vi "INIT.vi"(8 "error in (no error)":errorcluster, 11 "STREAK_camera in":refnum<class "STREAK_camera.lvclass">) -> (0 "error out":errorcluster, 3 "STREAK_camera out":refnum<class "STREAK_camera.lvclass">)   [LabVIEW 2019, in "STREAK_camera.lvclass"]
uses:
  STREAK_camera.lvclass
  Detector.lvclass
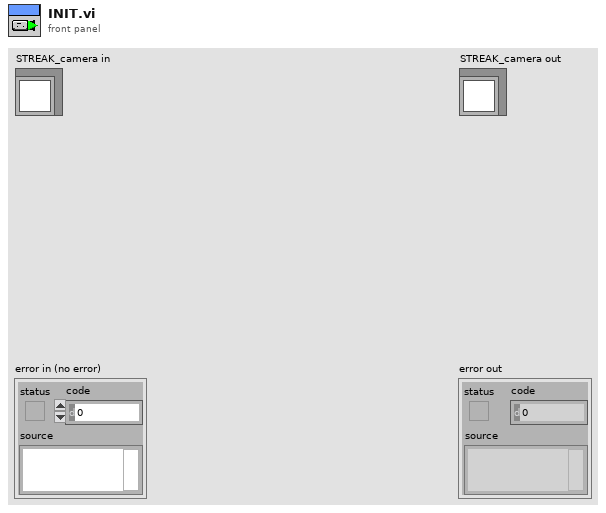
[diagram p1: front panel]
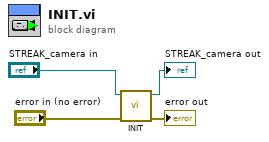
[diagram p0: block diagram]
diagram:
  n1 = call-parent "INIT.vi"("error in (no error)"="error in (no error)", "Detector in"="STREAK_camera in") -> ("error out"=→"error out":errorcluster, "Detector out"=→"STREAK_camera out":refnum<class "STREAK_camera.lvclass">)  [unwired: 8 in]
